vi "Path to Connection String.vi"(3 "Path":path) -> (1 "Connection String":string)   [LabVIEW 2011]
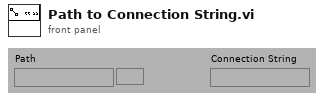
[diagram p1: front panel]
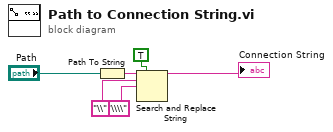
[diagram p0: block diagram]
diagram:
  n1 = Path To String(path="Path") -> (string=w3:string)
  n2 = Search and Replace String(replace all?=TRUE ("replace all? (F)"), input string=w3, search string="\\", replace string="\\\\" ("search string")) -> (result string=→"Connection String":string)  [unwired: 1 in, 6 out]
